vi "Execution Unit.Async.vi"(10 "Parameters":variant, 11 "Process":refnum<class "Process.lvclass">) -> ()   [LabVIEW 2020, in "AIM ARINC 429 Engine.lvlib" / "Custom Device.lvlib"]
uses:
  Custom Device.lvlib
  <vilib>/NI/NIVS Inline Async API/_VS Inline Async API/Process/Process.lvclass
  Asynchronous Process Parameters.ctl
  Asynchronous Execution Unit Runtime Information.ctl
  Interfaces/Execution Unit/Execution Unit.lvclass
  Interfaces/Shared Resources/Shared Resources.lvclass
  <vilib>/NI/NIVS Inline Async API/_VS Inline Async API/Process/Process.lvclass/Process.ctl
  <vilib>/NI/NIVS Inline Async API/_Data Access Engine/Access Type Classes/ReadWrite/ReadWrite.lvclass/ReadWrite.ctl
  <vilib>/NI/NIVS Inline Async API/_Data Access Engine/Access Type Classes/Read/Read.lvclass/Read.ctl
  <vilib>/NI/NIVS Inline Async API/_Data Access Engine/Access Type Classes/Write/Write.lvclass/Write.ctl
  <vilib>/NI/NIVS Inline Async API/_VS Inline Async API/Process/Data Member Access/Read Data Access.vi
  <vilib>/NI/NIVS Inline Async API/_VS Inline Async API/Error Handling Process/SubVIs/Error.ConvertArray.vi
  <vilib>/NI/NIVS Inline Async API/_Data Access Engine/Access Type Classes/Read/Read.ProcessData.vi
  <vilib>/NI/NIVS Inline Async API/_Data Access Engine/Access Type Classes/ReadWrite/ReadWrite.ProcessData.vi
  <vilib>/NI/NIVS Inline Async API/_Data Access Engine/Access Type Classes/Write/Write.ProcessData.vi
  <vilib>/NI/NIVS Inline Async API/_Data Access Engine/Access Type Classes/Write/Write.Buffer.vi
  <vilib>/NI/NIVS Inline Async API/_Data Access Engine/Access Type Classes/Write/Write.Commit.vi
  <vilib>/NI/NIVS Inline Async API/_Data Access Engine/Data Access Engine/Methods/Write.Lookup.vi
  <vilib>/NI/NIVS Inline Async API/_Data Access Engine/Data Access Engine/Methods/ReadWrite.Lookup.vi
  <vilib>/NI/NIVS Inline Async API/_Data Access Engine/Data Access Engine/Methods/Read.Lookup.vi
  <vilib>/NI/NIVS Inline Async API/_Data Access Engine/Data Access Engine/Data Access Engine.lvclass
  <vilib>/NI/NIVS Inline Async API/_Data Access Engine/Data Access Engine/Methods/ReadWrite.Data.vi
  <vilib>/NI/NIVS Inline Async API/_Data Access Engine/Data Access Engine/Methods/Write.Data.vi
  <vilib>/NI/NIVS Inline Async API/_Data Access Engine/Data Access Engine/Methods/Read.Data.vi
  <vilib>/NI/NIVS Inline Async API/_Data Access Engine/Access Type Classes/ReadWrite/ReadWrite.lvclass
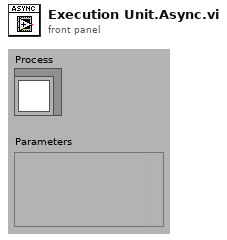
[diagram p1: front panel]
types:
  T1 = typedef "AIM ARINC 429 Engine.lvlib/Custom Device.lvlib/Asynchronous Process Parameters.ctl" = cluster{"Grouped Asynchronous Execution Unit Runtime Information":T2[], "shared resources":refnum<class "Shared Resources.lvclass">}
  T2 = typedef "AIM ARINC 429 Engine.lvlib/Custom Device.lvlib/Asynchronous Execution Unit Runtime Information.ctl" = cluster{"Execution Unit":refnum<class "Execution Unit.lvclass">, "Incoming Channel Group Name":string, "Outgoing Channel Group Name":string, "ReadWrite Channel Group Name":string}
  T3 = typedef "Data Access Engine.lvlib/Data Access Engine.lvclass/Write.DVR.ctl" = refnum<data-value>
  T4 = typedef "Data Access Engine.lvlib/Data Access Engine.lvclass/ReadWrite.DVR.ctl" = refnum<data-value>
  T5 = typedef "Data Access Engine.lvlib/Data Access Engine.lvclass/Read.DVR.ctl" = refnum<data-value>
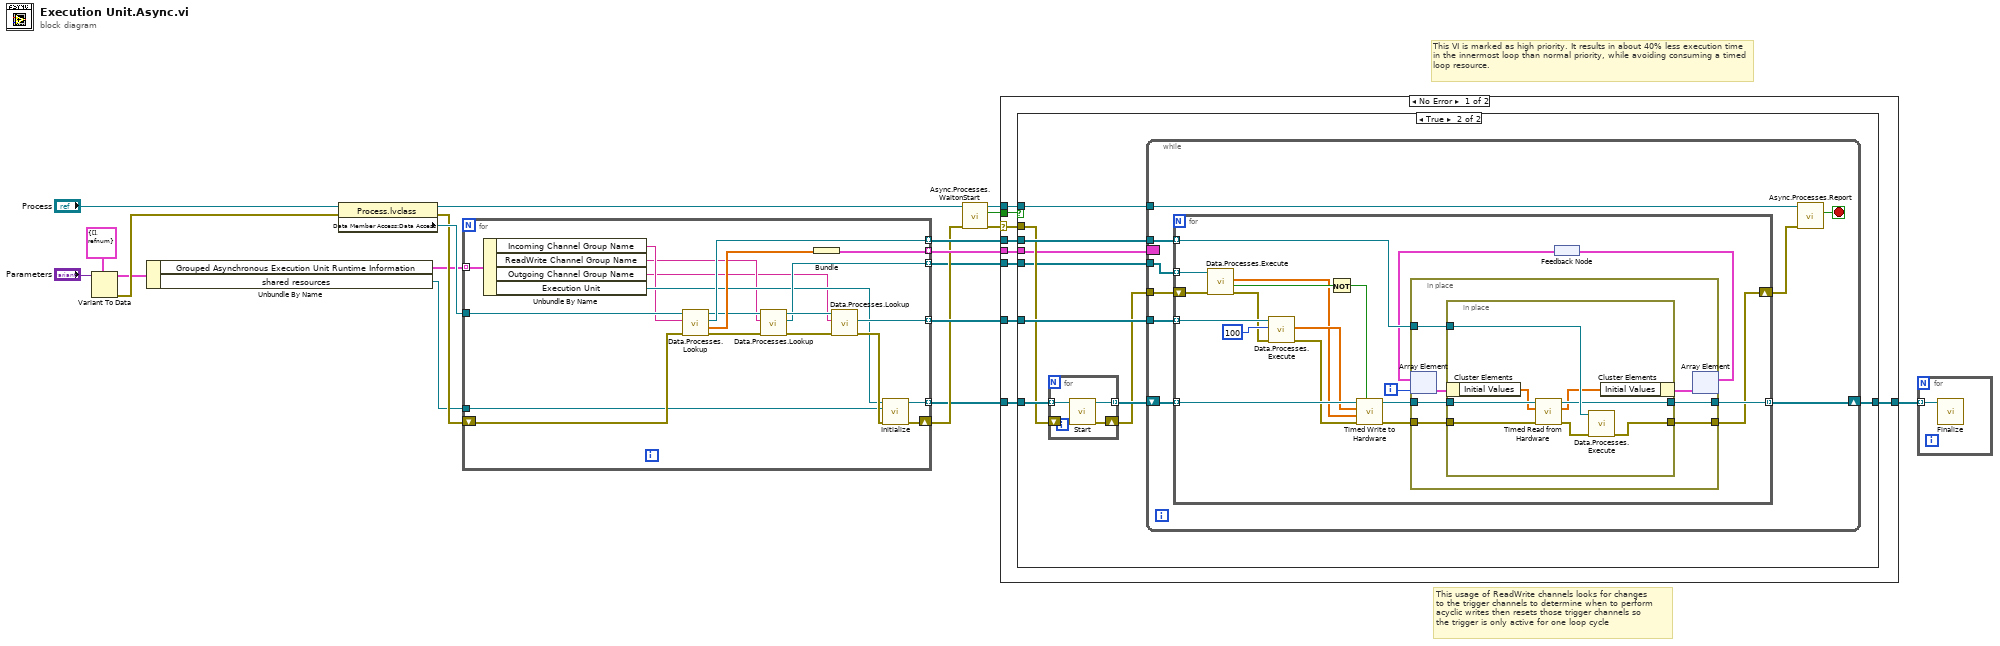
[diagram p0: block diagram]
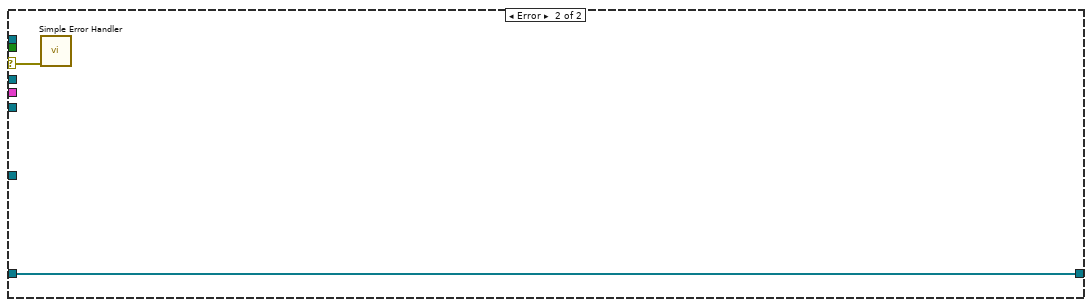
[diagram p3: hidden frame]
diagram:
  # "This VI is marked as high priority. It results in about 40% less execution time in the innermost loop than normal priority, while avoiding consuming a timed loop resource."
  # "This usage of ReadWrite channels looks for changes\nto the trigger channels to determine when to perform\nacyclic writes then resets those trigger channels so\nthe trigger is only active for one loop cycle"
  n1 = Variant To Data(type=T1 {"Grouped Asynchronous Execution Unit Runtime Information"=[], "shared resources"=refnum} ("Asynchronous Process Parameters"), Variant="Parameters") -> (data=w4:T1, error out=w9:errorcluster)  [unwired: 1 in]
  n2 = Unbundle By Name(w4) -> ("Grouped Asynchronous Execution Unit Runtime Information"=w2:T2[], "shared resources"=w3:refnum<class "Shared Resources.lvclass">)
  n3 = property class="Process.lvclass"(reference="Process", error in=w9) -> (reference out=w14:refnum<class "Process.lvclass">, error out=w12:errorcluster, "Data Member Access:Data Access"=w13:refnum<class "Data Access Engine.lvclass">)
  n4 = for {
    tunnel: [w40] -> w17 mode=indexing
    tunnel: [w39] -> w16 mode=indexing
    tunnel: w13 -> [w38]
    tunnel: [w25] -> w8 mode=indexing
    tunnel: [w31] -> w5 mode=indexing
    tunnel: w3 -> [w28]
    shift-right: [w34] -> w7
    shift-left: w12 -> [w37]
    tunnel: w2 -> [w27] mode=indexing
    tunnel: [w24] -> w1 mode=indexing
    n5 = Unbundle By Name(w27) -> ("Incoming Channel Group Name"=w23:string, "ReadWrite Channel Group Name"=w22:string, "Outgoing Channel Group Name"=w21:string, "Execution Unit"=w26:refnum<class "Execution Unit.lvclass">)
    n6 = call-poly <vilib>:"Data.Processes.Lookup.vi"("error in (no error)"=w37, "Name"=w23, "Data Access API in"=w38) -> ("error out"=w30:errorcluster, "Initial Values"=w36:dbl[], "Ref"=w39:T3, "Data Access API out"=w33:refnum<class "Data Access Engine.lvclass">)  [unwired: 5 in]
    n7 = call-poly <vilib>:"Data.Processes.Lookup.vi"("error in (no error)"=w30, "Name"=w22, "Data Access API in"=w33) -> ("error out"=w29:errorcluster, "Ref"=w31:T4, "Data Access API out"=w32:refnum<class "Data Access Engine.lvclass">)  [unwired: 5 in, 1 out]
    n8 = Bundle("Initial Values"=w36) -> (w25:cluster{"Initial Values":dbl[]})  [unwired: 1 in]
    n9 = call-poly <vilib>:"Data.Processes.Lookup.vi"("error in (no error)"=w29, "Name"=w21, "Data Access API in"=w32) -> ("error out"=w35:errorcluster, "Ref"=w40:T5)  [unwired: 5 in, 2 out]
    n10 = call-dynamic "Initialize.vi"("error in (no error)"=w35, "shared resources"=w28, "Execution Unit in"=w26) -> ("error out"=w34:errorcluster, "Execution Unit out"=w24:refnum<class "Execution Unit.lvclass">)  [unwired: 7 in]
  }
  n11 = call <vilib>:"Async.Processes.WaitonStart.vi"("error in (no error)"=w7, "Process"=w14) -> ("error out"=w18:errorcluster, "Execute"=w20:bool, "Process out"=w19:refnum<class "Process.lvclass">)  [unwired: 7 in]
  n12 = case shown="No Error" w18 {
    selector: w18 -> [w45 w109]
    tunnel: w20 -> [w49 _]
    tunnel: w19 -> [w48 _]
    tunnel: w16 -> [w47 _]
    tunnel: w17 -> [w46 _]
    tunnel: w8 -> [w44 _]
    tunnel: w1 -> [w43 w108]
    tunnel: [w42 w108] -> w6
    tunnel: w5 -> [w41 _]
    frame No Error {
      n13 = case shown="True" w49 {
        tunnel: w45 -> [_ w56]
        tunnel: w48 -> [_ w58]
        tunnel: w46 -> [_ w60]
        tunnel: w47 -> [_ w59]
        tunnel: w44 -> [_ w55]
        tunnel: w43 -> [w50 w57]
        tunnel: [w50 w54] -> w42
        tunnel: w41 -> [_ w53]
        frame False {
        }
        frame True {
          n14 = for {
            tunnel: w57 -> [w107] mode=indexing
            tunnel: [w105] -> w52 mode=indexing
            shift-right: [w104] -> w51
            shift-left: w56 -> [w106]
            n15 = call-dynamic "Start.vi"("error in (no error)"=w106, "Execution Unit in"=w107) -> ("error out"=w104:errorcluster, "Execution Unit out"=w105:refnum<class "Execution Unit.lvclass">)  [unwired: 8 in]
          }
          n16 = while {
            tunnel: w58 -> [w69]
            tunnel: w60 -> [w67]
            tunnel: w59 -> [w66]
            border: w55 -> [_]
            shift-right: [w63] -> w54
            shift-left: w52 -> [w65]
            tunnel: w53 -> [w61]
            tunnel: w51 -> [w62]
            stop <- w68 stop-if-true
            n17 = for {
              tunnel: w67 -> [w88] mode=indexing
              tunnel: w66 -> [w79] mode=indexing
              tunnel: w65 -> [w73] mode=indexing
              tunnel: [w86] -> w63 mode=indexing
              tunnel: w61 -> [w85] mode=indexing
              shift-right: [w80] -> w64
              shift-left: w62 -> [w84]
              i -> [w81]
              n18 = call-poly <vilib>:"Data.Processes.Execute.vi"("error in (no error)"=w84, "Ref"=w85) -> ("error out"=w83:errorcluster, "Timeout?"=w82:bool, "Data"=w70:dbl[])  [unwired: 6 in, 1 out]
              n19 = call-poly <vilib>:"Data.Processes.Execute.vi"("error in (no error)"=w83, "timeout ms"=100, "Ref"=w88) -> ("error out"=w72:errorcluster, "Values"=w71:dbl[])  [unwired: 6 in, 1 out]
              n20 = Not(x=w82) -> (.not. x?=w74:bool)
              n21 = call "Timed Write to Hardware.vi"("Valid"=w74, "error in (no error)"=w72, "Trigger Values"=w70, "Values"=w71, "Execution Unit in"=w73) -> ("error out"=w77:errorcluster, "Execution Unit out"=w78:refnum<class "Execution Unit.lvclass">)  [unwired: 3 in, 2 out]
              n22 = feedback #1() -> (w76:cluster{"Initial Values":dbl[]}[])
              n23 = in-place {
                in-place-border: w78 -> [w95]
                in-place-border: [w94] -> w80
                in-place-border: [w93] -> w86
                in-place-border: w77 -> [w92]
                in-place-border: w79 -> [w90]
                n24 = in-place-array #2(w76, w81) -> (w91:cluster{"Initial Values":dbl[]})
                n25 = in-place {
                  in-place-border: w95 -> [w99]
                  in-place-border: [w102] -> w94
                  in-place-border: [w100] -> w93
                  in-place-border: w92 -> [w98]
                  in-place-border: w90 -> [w101]
                  n26 = in-place-cluster #3(w91) -> ("Initial Values"=w97:dbl[])
                  n27 = call "Timed Read from Hardware.vi"("error in"=w98, "Values in"=w97, "Execution Unit in"=w99) -> ("error out"=w103:errorcluster, "Values out"=w96:dbl[], "Execution Unit out"=w100:refnum<class "Execution Unit.lvclass">)  [unwired: 6 in]
                  n28 = call-poly <vilib>:"Data.Processes.Execute.vi"("error in (no error)"=w103, "Ref"=w101) -> ("error out"=w102:errorcluster)  [unwired: 9 in]
                  n29 = in-place-cluster #3("Initial Values"=w96) -> (w89:cluster{"Initial Values":dbl[]})
                }
                n30 = in-place-array #2(w89) -> (w75:cluster{"Initial Values":dbl[]}[])  [unwired: 1 out]
              }
              n31 = feedback-in #1(w75) -> ()
            }
            n32 = call <vilib>:"Async.Processes.Report.vi"("Error"=w64, "Process in"=w69) -> ("Stop"=w68:bool)  [unwired: 8 in, 1 out]
          }
        }
      }
    }
    frame Error {
      n33 = call <vilib>:"Simple Error Handler.vi"("error in (no error)"=w109) -> ()  [unwired: 4 in, 5 out]
    }
  }
  n34 = for {
    tunnel: w6 -> [w110] mode=indexing
    n35 = call-dynamic "Finalize.vi"("Execution Unit in"=w110) -> ()  [unwired: 9 in, 2 out]
  }
